vi "Get Notification Map.vi"(8 "error in (no error)":errorcluster, 11 "TwinCAT ADS in":refnum<class "TwinCAT ADS.lvclass">) -> (0 "error out":errorcluster, 2 "Notification Map":refnum<data-value>, 3 "TwinCAT ADS out":refnum<class "TwinCAT ADS.lvclass">)   [LabVIEW 2018, in "TwinCAT ADS.lvclass"]
uses:
  TwinCAT ADS.lvclass
  TwinCAT ADS.lvclass/TwinCAT ADS.ctl
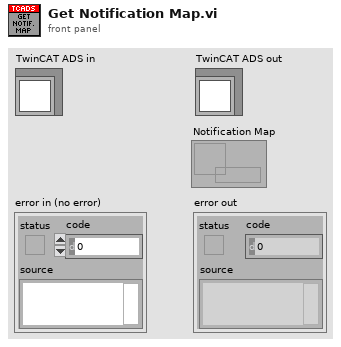
[diagram p1: front panel]
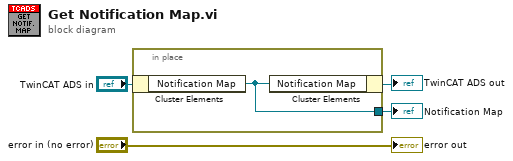
[diagram p0: block diagram]
diagram:
  n1 = in-place {
    in-place-border: [w5] -> w1
    n2 = in-place-cluster #1("TwinCAT ADS in") -> ("Notification Map"=w5:refnum<data-value>)
    n3 = in-place-cluster #1("Notification Map"=w5) -> (→"TwinCAT ADS out":refnum<class "TwinCAT ADS.lvclass">)
  }
  "Notification Map" <- w1
  "error out" <- "error in (no error)"
